vi "Test C.vi"(8 "error in (no error)":errorcluster) -> (0 "error out":errorcluster)   [LabVIEW 2019, in "Sequence Example.lvlib"]
uses:
  Sequence Example.lvlib
  b65cedc0-6f88-47fe-863c-f92be18f8f6a.vi
  f0c8a91b-42a2-41e7-93a8-f572df4bd512.vi
  LVUT Global 1.vi
  <vilib>/Utility/Data Type/Get Type Information.vi
  <vilib>/Utility/error.llb/Trim Whitespace.vi
  Equal Value.vi
  Unit Test Engine Tools.lvlib
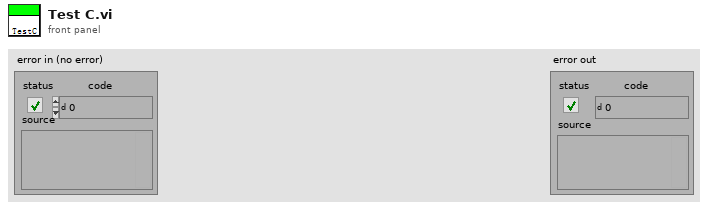
[diagram p1: front panel]
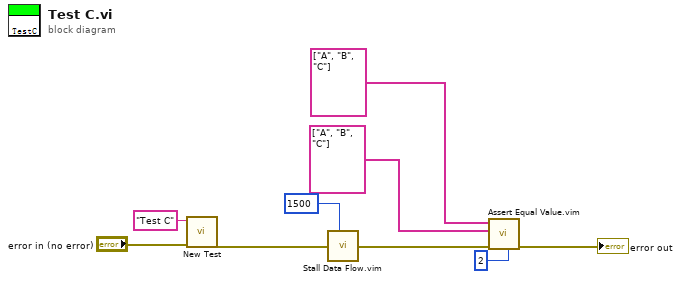
[diagram p0: block diagram]
diagram:
  n1 = call "New Test.vi"("error in (no error)"="error in (no error)", "Test"="Test C") -> ("error out"=w7:errorcluster)  [unwired: 9 in]
  n2 = call "Stall Data Flow.vim"("value in"=w7, "milliseconds to wait"=u32 1500) -> ("value out"=w4:errorcluster)  [unwired: 1 out]
  n3 = call "Assert Equal Value.vim"("precision (6)"=i16 2, "error in (no error)"=w4, "Y"=string[] ["A", "B", "C"], "X"=string[] ["A", "B", "C"]) -> ("error out"=→"error out":errorcluster)  [unwired: 7 in]
